vi "FromData.vi"(8 "error in (no error)":errorcluster, 10 "Data":string, 11 "E55555 in":refnum<class "E55555.lvclass">) -> (0 "error out":errorcluster, 3 "E55555 out":refnum<class "Error.lvclass">)   [LabVIEW 2022 SP3, in "Demo.lvlib" / "E55555.lvclass"]
uses:
  E55555.lvclass
  C:/Users/jakub/repos/gh/lv-error/Source/Error/Error/Error.lvclass
  Error/Error/Error.lvclass
  E55555.lvclass/E55555.ctl
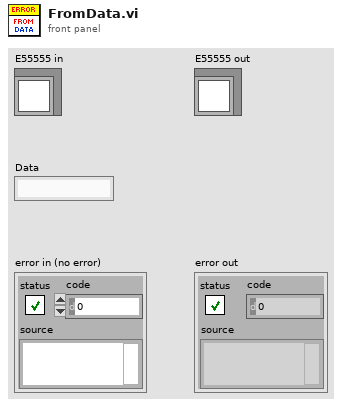
[diagram p1: front panel]
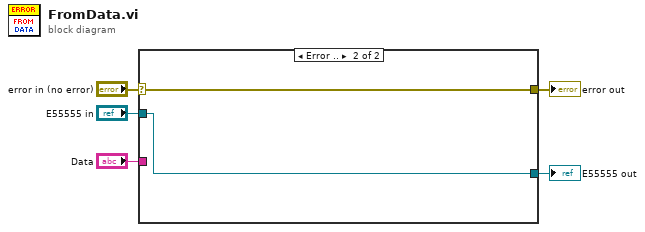
[diagram p0: block diagram]
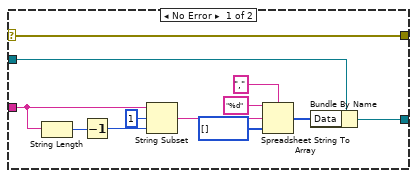
[diagram p2: hidden frame]
diagram:
  n1 = case shown="Error .." "error in (no error)" {
    selector: "error in (no error)" -> [w13 w19]
    tunnel: [w13 w19] -> w5
    tunnel: [w7 w18] -> w4
    tunnel: "Data" -> [w16 _]
    tunnel: "E55555 in" -> [w6 w18]
    frame No Error {
      n2 = String Length(string=w16) -> (length=w15:i32)
      n3 = Decrement(x=w15) -> (x-1=w14:i32)
      n4 = String Subset(string=w16, offset (0)=1, length (rest)=w14) -> (substring=w12:string)
      n5 = Spreadsheet String To Array(delimiter (Tab)=",", format string="%d", spreadsheet string=w12, array type (2D Dbl)=i32[] []) -> (array=w8:i32[])
      n6 = Bundle By Name(cluster=w6, "Data"=w8) -> (w7:refnum<class "E55555.lvclass">)
    }
    frame Error {
    }
  }
  "error out" <- w5
  "E55555 out" <- w4
